vi "integral_of_2.15_m.vi"(0 "u*":dbl format="%.2f", 2 "v*":dbl format="%.2f", 3 "grid size for z*":i16, 4 "Initialise":bool) -> (5 "p(u*,v*)":dbl format="%.2f")   [LabVIEW 2010]
uses:
  xw_correction_global_m.vi
  <vilib>/Analysis/NI_AALPro.lvlib
panel:
  out "omega0":dbl format="%.5f"
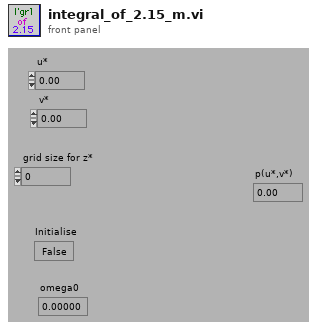
[diagram p1: front panel]
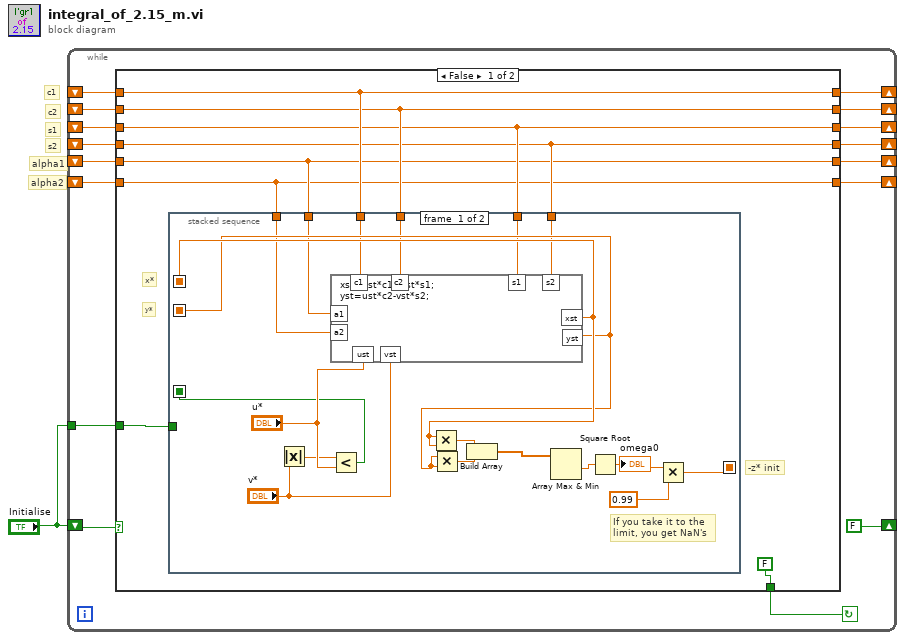
[diagram p0: block diagram]
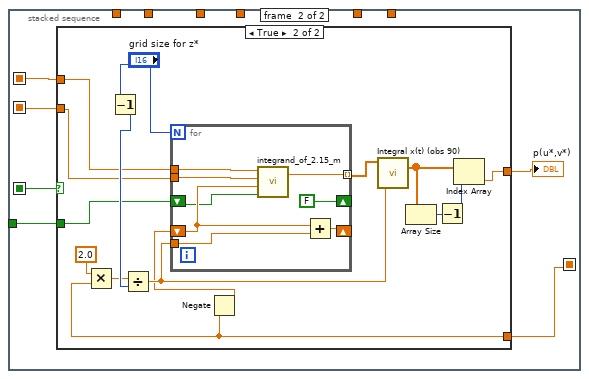
[diagram p2: hidden frame]
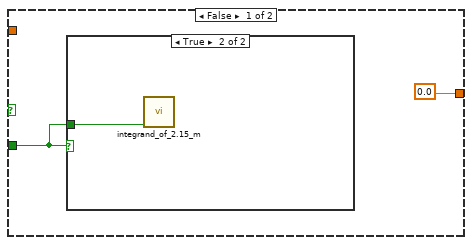
[diagram p3: hidden frame]
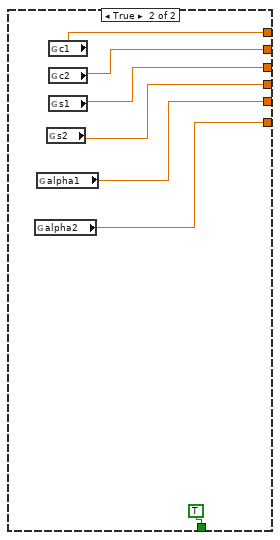
[diagram p5: hidden frame]
diagram:
  # "alpha2"
  # "alpha1"
  # "s2"
  # "s1"
  # "c2"
  # "c1"
  n1 = while {
    shift-left: _ -> [w12]
    shift-right: [w4] -> _
    shift-left: _ -> [w13]
    shift-right: [w5] -> _
    shift-left: _ -> [w2]
    shift-right: [w6] -> _
    shift-left: _ -> [w3]
    shift-right: [w7] -> _
    shift-left: _ -> [w10]
    shift-right: [w8] -> _
    shift-left: _ -> [w11]
    shift-right: [w9] -> _
    tunnel: "Initialise" -> [w14]
    shift-left: "Initialise" -> [w15]
    shift-right: [FALSE] -> _
    stop <- w17 continue-if-true
    n2 = case shown="False" w15 {
      tunnel: [FALSE TRUE] -> w17
      tunnel: w14 -> [w24 _]
      tunnel: w13 -> [w19 _]
      tunnel: w12 -> [w18 _]
      tunnel: w11 -> [w23 _]
      tunnel: w10 -> [w22 _]
      tunnel: [w23 w83] -> w9
      tunnel: [w22 w82] -> w8
      tunnel: [w21 w81] -> w7
      tunnel: [w20 w80] -> w6
      tunnel: [w19 w79] -> w5
      tunnel: [w18 w78] -> w4
      tunnel: w3 -> [w21 _]
      tunnel: w2 -> [w20 _]
      frame False {
        # "-z* init"
        # "y*"
        # "x*"
        n3 = stacked-sequence {
          seq-local: [w42 _] -> [_ w48]
          seq-local: [w34 _] -> [_ w50]
          seq-local: [w33 _] -> [_ w49]
          seq-local: [w35 _] -> [_ w46]
          tunnel: w24 -> [_ w45]
          tunnel: w19 -> [w31 _]
          tunnel: w18 -> [w30 _]
          tunnel: w23 -> [w29 _]
          tunnel: w22 -> [w28 _]
          tunnel: w21 -> [w27 _]
          tunnel: w20 -> [w26 _]
          frame #0 {
            # "If you take it to the \nlimit, you get NaN's"
            n4 = Absolute Value(x="v*") -> (abs(x)=w36:dbl)
            n5 = formula code="xst=ust*c1+vst*s1;\nyst=ust*c2-vst*s2;"("a1"=w31, "a2"=w30, "ust"="u*", "vst"="v*", "c1"=w29, "c2"=w28, "s1"=w27, "s2"=w26) -> ("xst"=w34:dbl, "yst"=w33:dbl)
            n6 = Less?(x=w36, y="u*") -> (x < y?=w35:bool)
            n7 = Multiply(x=w34, y=w34) -> (x*y=w39:dbl)
            n8 = Multiply(x=w33, y=w33) -> (x*y=w40:dbl)
            n9 = Build Array(w39, w40) -> (w32:dbl[])
            n10 = Array Max & Min(array=w32) -> (min value=w44:dbl)  [unwired: 3 out]
            n11 = Square Root(x=w44) -> (sqrt(x)=w43:dbl)
            "omega0" <- w43
            n12 = Multiply(x=w43, y=0.99) -> (x*y=w42:dbl)
          }
          frame #1 {
            n13 = case shown="True" w46 {
              tunnel: [0.0 w59] -> w47
              tunnel: w48 -> [_ w58]
              tunnel: w49 -> [_ w57]
              tunnel: w50 -> [_ w56]
              tunnel: w45 -> [w51 w54]
              frame False {
                n14 = case shown="True" w51 {
                  tunnel: w51 -> [_ w53]
                  frame False {
                  }
                  frame True {
                    n15 = call "integrand_of_2.15_m.vi"("Initialise"=w53) -> ()  [unwired: 3 in, 1 out]
                  }
                }
              }
              frame True {
                n16 = Multiply(x=2.0, y=w58) -> (x*y=w64:dbl)
                n17 = Decrement(x="grid size for z*") -> (x-1=w68:i16)
                n18 = Divide(x=w64, y=w68) -> (x/y=w66:dbl)
                n19 = Negate(x=w58) -> (-x=w55:dbl)
                n20 = for {
                  N: "grid size for z*" -> [_]
                  tunnel: w56 -> [w76]
                  tunnel: w57 -> [w75]
                  tunnel: w66 -> [w71]
                  tunnel: [w74] -> w65 mode=indexing
                  shift-right: [w73] -> _
                  shift-left: w55 -> [w72]
                  shift-right: [FALSE] -> _
                  shift-left: w54 -> [w70]
                  n21 = call "integrand_of_2.15_m.vi"("Initialise"=w70, "z*"=w72, "y*"=w75, "x*"=w76) -> ("Integrand"=w74:dbl)
                  n22 = Add(x=w72, y=w71) -> (x+y=w73:dbl)
                }
                n23 = call <vilib>:"Integral x(t) (obs 90).vi"("dt"=w66, "X"=w65) -> ("Integral X"=w62:dbl[])  [unwired: 2 in, 1 out]
                n24 = Array Size(array=w62) -> (size(s)=w61:i32)
                n25 = Decrement(x=w61) -> (x-1=w67:i32)
                n26 = Index Array(array=w62, index=w67) -> (element=w59:dbl)
              }
            }
            "p(u*,v*)" <- w47
          }
        }
      }
      frame True {
        n27 = global read "xw_correction_global_m.vi" "alpha2"() -> (w78:dbl)
        n28 = global read "xw_correction_global_m.vi" "alpha1"() -> (w79:dbl)
        n29 = global read "xw_correction_global_m.vi" "s2"() -> (w80:dbl)
        n30 = global read "xw_correction_global_m.vi" "c1"() -> (w83:dbl)
        n31 = global read "xw_correction_global_m.vi" "c2"() -> (w82:dbl)
        n32 = global read "xw_correction_global_m.vi" "s1"() -> (w81:dbl)
      }
    }
  }
